vi "Untitled 1.vi"() -> ()   [LabVIEW 2013]
uses:
  <vilib>/Instr/_visa.llb/VISA Configure Serial Port (Instr).vi
panel:
  out "Waveform Chart":u8[](graph)
  out "unsigned byte array":u8[](array[numeric])
  in  "parity (0:none)":enum16{"None", "Odd", "Even", "Mark", "Space"}(ring)
  in  "data bits (8)":u16=8 min=5 max=8 step=1
  out "read buffer":string
  in  "baud rate":u32=9600
  in  "VISA resource name":refnum<visa-resource-name>
  in  "stop":bool
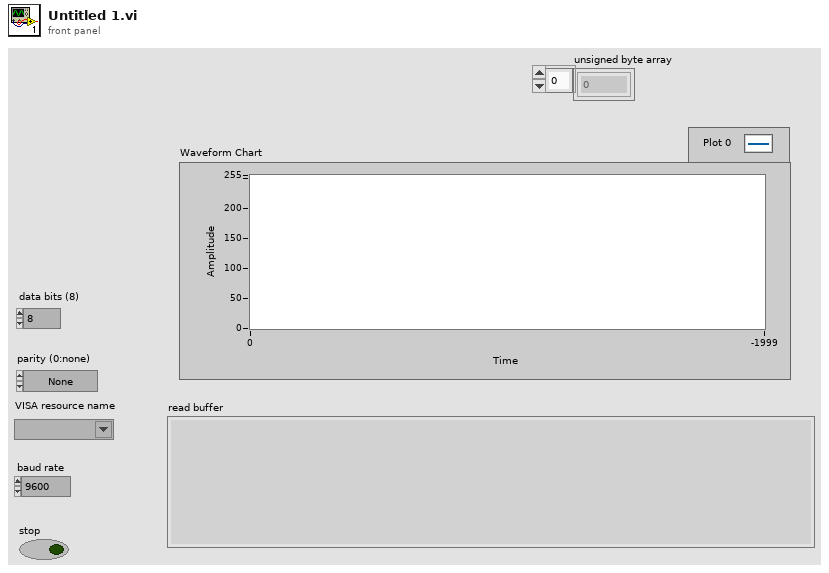
[diagram p1: front panel]
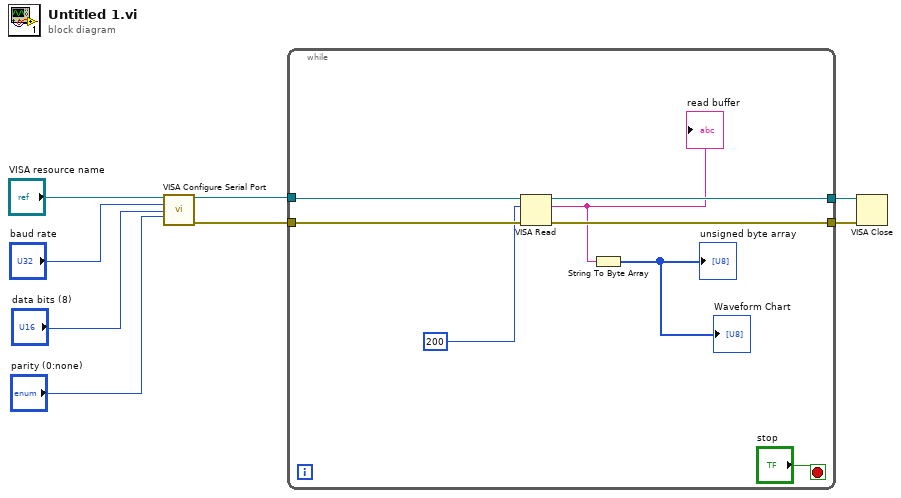
[diagram p0: block diagram]
diagram:
  n1 = call-poly "VISA Configure Serial Port"("VISA resource name"="VISA resource name", "baud rate (9600)"="baud rate", "data bits (8)"="data bits (8)", "parity (0:none)"="parity (0:none)") -> ("VISA resource name out"=w8:refnum<visa-resource-name>, "error out"=w6:errorcluster)  [unwired: 10 in]
  n2 = while {
    tunnel: w8 -> [w13]
    tunnel: [w15] -> w7
    tunnel: w6 -> [w12]
    tunnel: [w14] -> w5
    stop <- "stop" stop-if-true
    n3 = VISA Read(VISA resource name=w13, byte count=u32 200, error in (no error)=w12) -> (VISA resource name out=w15:refnum<visa-resource-name>, read buffer=w10:string, error out=w14:errorcluster)  [unwired: 1 out]
    "read buffer" <- w10
    n4 = String To Byte Array(string=w10) -> (unsigned byte array=→"unsigned byte array" →"Waveform Chart":u8[])
  }
  n5 = VISA Close(VISA resource name=w7, error in (no error)=w5) -> ()  [unwired: 1 out]
